vi "test chillhub serial.vi"() -> ()   [LabVIEW 2012]
uses:
  <vilib>/Instr/_visa.llb/VISA Configure Serial Port (Instr).vi
panel:
  out "read buffer 2":string
  out "write buffer":string
  out "read buffer":string
  in  "stop":bool
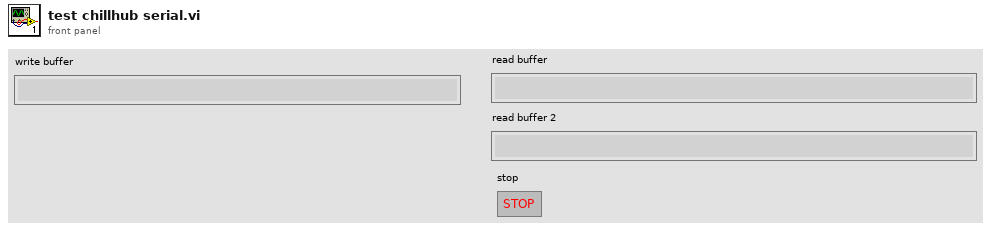
[diagram p1: front panel]
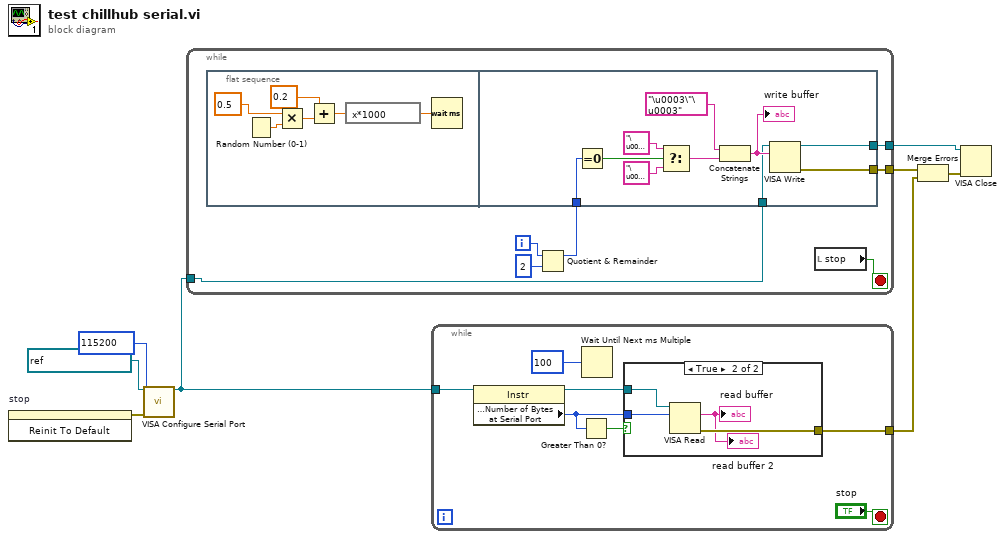
[diagram p0: block diagram]
diagram:
  n1 = invoke on="stop" class="Bool (strict)" method="Reinit To Default"() -> (error out=w2:errorcluster)  [unwired: 3 in, 2 out]
  n2 = call-poly "VISA Configure Serial Port"("VISA resource name"=refnum<visa-resource-name> "COM13", "baud rate (9600)"=u32 115200, "error in (no error)"=w2) -> ("VISA resource name out"=w6:refnum<visa-resource-name>)  [unwired: 11 in, 1 out]
  n3 = while {
    tunnel: [w11] -> w7
    tunnel: w6 -> [w10]
    tunnel: [w9] -> w5
    i -> [w14]
    stop <- w15 stop-if-true
    n4 = flat-sequence {
      tunnel: w12 -> [w28]
      tunnel: [w24] -> w11
      tunnel: w10 -> [w23]
      tunnel: [w22] -> w9
      frame #0 {
        n5 = Random Number (0-1)() -> (number: 0 to 1=w21:dbl)
        n6 = Multiply(x=0.5, y=w21) -> (x*y=w20:dbl)
        n7 = Add(x=0.2, y=w20) -> (x+y=w19:dbl)
        n8 = expression code="x*1000"(w19) -> (w18:dbl)
        n9 = Wait (ms)(milliseconds to wait=w18) -> ()  [unwired: 1 out]
      }
      frame #1 {
        n10 = Equal To 0?(x=w28) -> (x = 0?=w27:bool)
        n11 = Select(t="\u0000" ("write buffer"), s=w27, f="\u0011" ("write buffer")) -> (s? t:f=w30:string)
        n12 = Concatenate Strings("\u0003\"\u0003" ("write buffer"), w30) -> (w29:string)
        "write buffer" <- w29
        n13 = VISA Write(VISA resource name=w23, write buffer=w29) -> (VISA resource name out=w24:refnum<visa-resource-name>, error out=w22:errorcluster)  [unwired: 1 in, 1 out]
      }
    }
    n14 = Quotient & Remainder(x=w14, y=2) -> (x-y*floor(x/y)=w12:i32)  [unwired: 1 out]
    n15 = local read "stop"() -> (w15:bool)
  }
  n16 = while {
    tunnel: w6 -> [w37]
    tunnel: [w33] -> w4
    stop <- "stop" stop-if-true
    n17 = property class="Instr"(reference=w37) -> (reference out=w36:refnum<visa-resource-name>, "Serial Settings:Number of Bytes at Serial Port"=w34:u32)  [unwired: 1 in, 1 out]
    n18 = Greater Than 0?(x=w34) -> (x > 0?=w35:bool)
    n19 = Wait Until Next ms Multiple(millisecond multiple=u32 100) -> ()  [unwired: 1 out]
    n20 = case shown="True" w35 {
      tunnel: w36 -> [_ w42]
      tunnel: w34 -> [_ w41]
      tunnel: [_ w40] -> w33
      frame False {
      }
      frame True {
        n21 = VISA Read(VISA resource name=w42, byte count=w41) -> (read buffer=→"read buffer" →"read buffer 2":string, error out=w40:errorcluster)  [unwired: 1 in, 2 out]
      }
    }
  }
  n22 = Merge Errors(w5, w4) -> (w3:errorcluster)
  n23 = VISA Close(VISA resource name=w7, error in (no error)=w3) -> ()  [unwired: 1 out]
